vi "ScanMode.vi"() -> ()   [LabVIEW 2014]
uses:
  ScanDM.ctl
  MetricControl.ctl
  Scan Metric.ctl
  <vilib>/Analysis/6fits.llb/Curve Fitting Criteria.ctl
  ScanEngineState.ctl
  <vilib>/Utility/miscctls.llb/LVPointDoubleTypeDef.ctl
  <vilib>/Analysis/NI_AALPro.lvlib
  <vilib>/gmath/NI_Gmath.lvlib
panel:
  in  "parameter bounds":T1={"amp min"=-inf, "amp max"=inf, "center min"=-inf, "center max"=inf, "deviation min"=-inf, "deviation max"=inf, "offset min"=0.0, "offset max"=0.0}
  in  "tolerance":dbl=0.0001 format="%#_3g"
  out "Best Gaussian Fit":dbl[](array[numeric])
  in  "method":T2 items=["Least Square", "Least Absolute Residual", "Bisquare"]
  in  "Manual Initial Guess":bool
  in  "Initial Guess":T3={"initial amplitude"=nan, "initial center"=nan, "initial standard deviation"=nan, "offset"=nan}
  in  "Fit Type":enum32{"Guass Fit", "Quad Fit"}(radio)
  out "Intensity Graph":sgl[][](graph)
  in  "Apply":bool
  in  "Find peak":bool
  in  "Cancel":bool
  in  "Metric Control":T4={"Use Metric"=FALSE, "DM Metric"=enum."No Zero Mean", "Smooth"=FALSE, "Pixels"=0.0, "ROI"=FALSE, "ROI Size"=0.0}
  in  "stop":bool
  out "Metric Display":cluster{"Amplititude":dbl[], "Metric":sgl[]}[](graph)
  in  "Scan Control":T6 {"Mode" items=["1", "2", "3", "4", "5", "6", "7", "8", "9", "10", "11", "12", "13", "14", "15", "16", "17", "18", "19", "20", "21", "22", "23", "24", "25", "26", "27", "28", "29", "30", "31", "32", "33", "34", "35", "36", "37", "38", "39", "40", "41", "42", "43", "44", "45", "46", "47", "48", "49", "50", "51", "52", "53", "54", "55", "56", "57", "58", "59", "60", "61", "62", "63", "64", "65", "66", "67", "68", "69", "70", "71", "72", "73", "74", "75", "76", "77", "78", "79", "80", "81", "82", "83", "84", "85", "86", "87", "88", "89", "90", "91", "92", "93", "94", "95", "96", "97", "98", "99", "100", "101", "102", "103", "104", "105", "106", "107", "108", "109", "110", "111", "112", "113", "114", "115", "116", "117", "118", "119", "120", "121", "122", "123", "124", "125", "126", "127", "128", "129", "130", "131", "132", "133", "134", "135", "136", "137", "138", "139", "140"]}
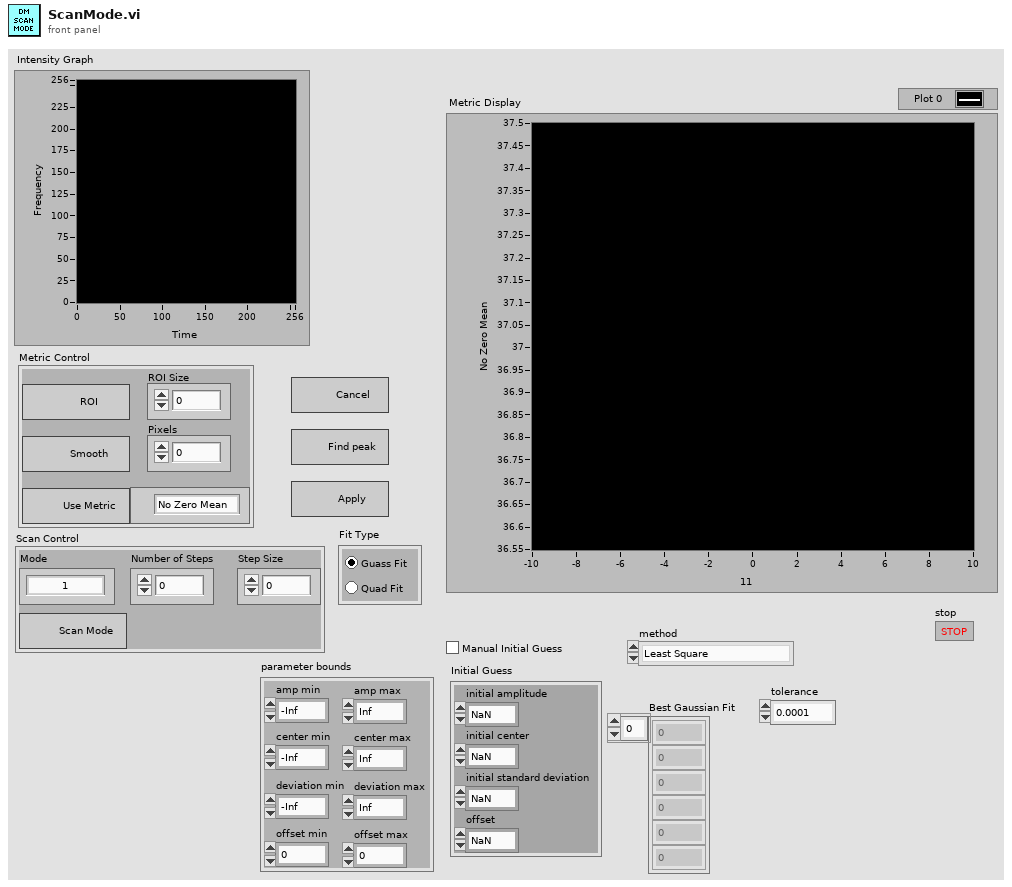
[diagram p1: front panel]
types:
  T1 = cluster{"amp min":dbl, "amp max":dbl, "center min":dbl, "center max":dbl, "deviation min":dbl, "deviation max":dbl, "offset min":dbl, "offset max":dbl}
  T2 = typedef "NI_AALPro.lvlib/Curve Fitting Criteria.ctl" = u16
  T3 = cluster{"initial amplitude":dbl, "initial center":dbl, "initial standard deviation":dbl, "offset":dbl}
  T4 = typedef "MetricControl.ctl" = cluster{"Use Metric":bool, "DM Metric":T5, "Smooth":bool, "Pixels":dbl, "ROI":bool, "ROI Size":dbl}
  T5 = typedef "Scan Metric.ctl" = enum16{"Max Intensity", "No Zero Mean", "Threshold"}
  T6 = typedef "ScanDM.ctl" = cluster{"Scan":bool, "Mode":u16, "Number of Steps":u8, "Step Size":dbl}
  T7 = typedef "ScanEngineState.ctl" = enum16{"DM_WRITE", "IMAGE", ""}
  T8 = typedef "LVPointDoubleTypeDef.ctl" = cluster{"X":dbl, "Y":dbl}
  T9 = enum16{"Linear", "Polynomial", "Exponential", "Power"}
  T10 = typedef "DMControl_STED.ctl" = cluster{"Type":enum32{"Mirror", "Abberation"}, "Modes":cluster{"Mode":string, "Amplititude":dbl}[], "Apply Flat":bool, "Save Map":bool, "Clear Voltage":bool, "Abberation Files":u16, "Scan ":bool}
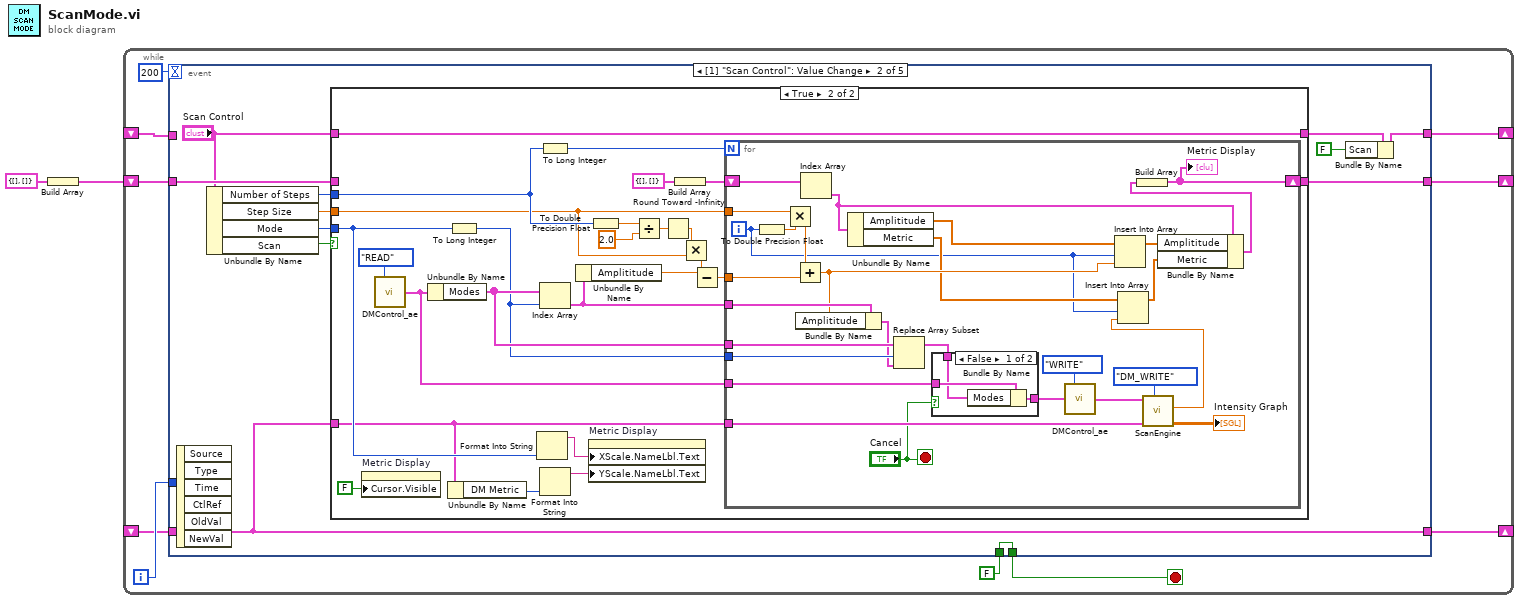
[diagram p0: block diagram]
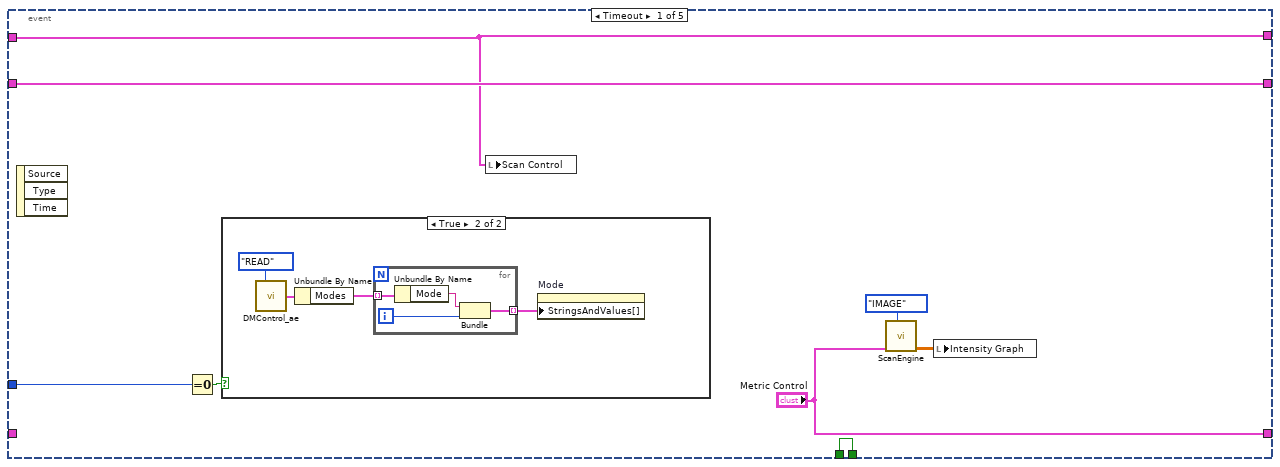
[diagram p2: hidden frame]
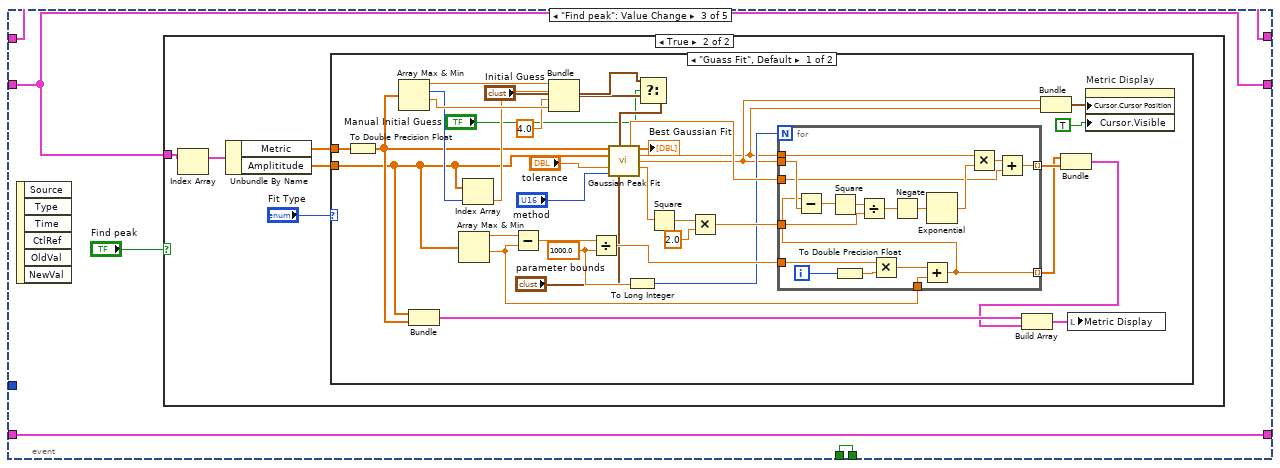
[diagram p6: hidden frame]
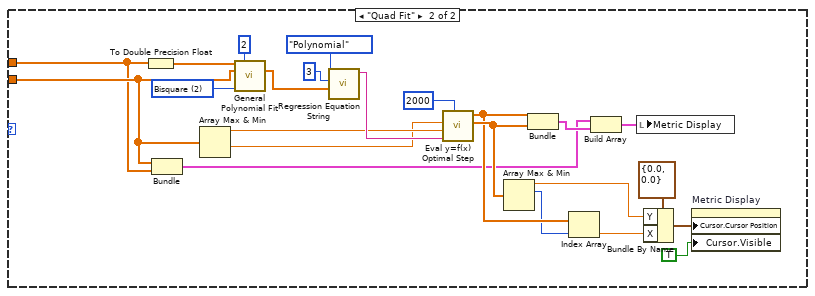
[diagram p8: hidden frame]
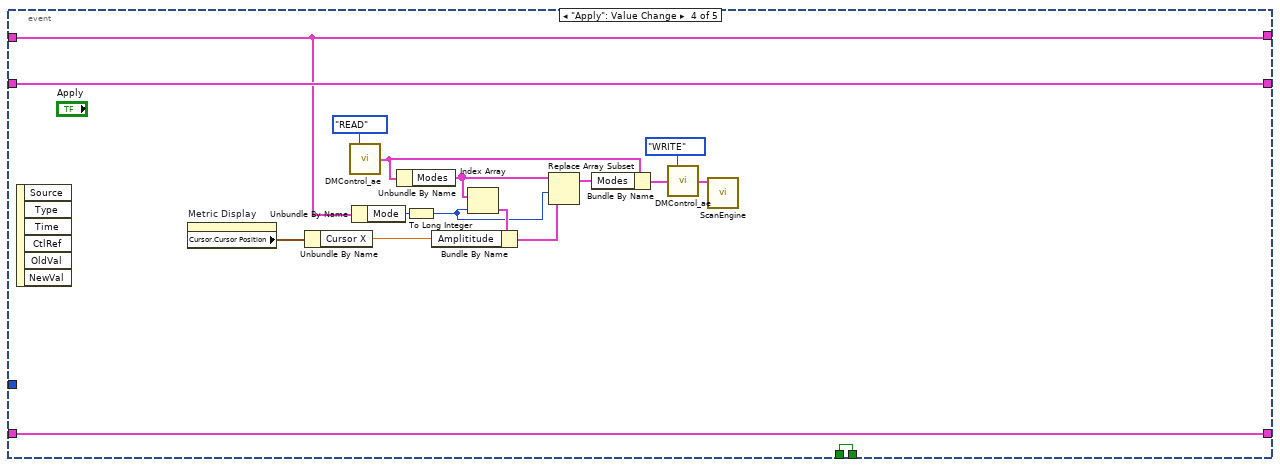
[diagram p9: hidden frame]
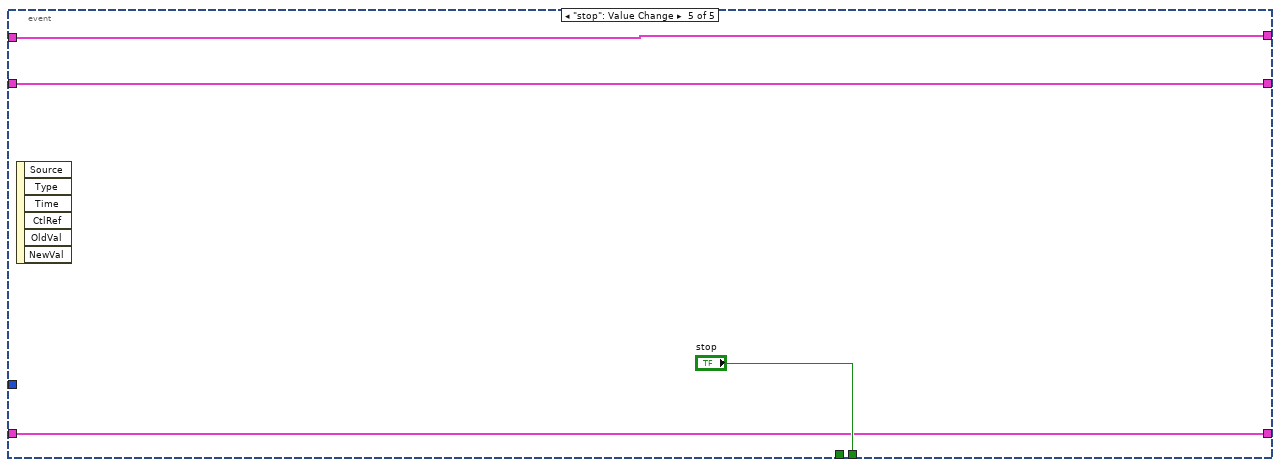
[diagram p10: hidden frame]
diagram:
  n1 = Build Array(cluster{"Amplititude":dbl[], "Metric":sgl[]} {"Amplititude"=[], "Metric"=[]} ("output cluster")) -> (w1:cluster{"Amplititude":dbl[], "Metric":sgl[]}[])
  n2 = while {
    shift-right: [w8] -> _
    shift-left: _ -> [w7]
    shift-right: [w6] -> _
    shift-left: w1 -> [w5]
    shift-right: [w3] -> _
    shift-left: _ -> [w4]
    i -> [w9]
    stop <- w12 stop-if-true
    n3 = event shown="[1] \"Scan Control\": Value Change" {
      selector: _ -> [_ _ _ _ _]
      dyn-events: _ -> [_ _ _ _ _]
      timeout: 200 -> [_ _ _ _ _]
      tunnel: [w20 w38 w101 w187 "stop"] -> w12
      tunnel: FALSE -> [w20 w38 w101 w187 _]
      tunnel: w9 -> [w18 _ _ _ _]
      tunnel: [w16 w30 w104 w198 w205] -> w8
      tunnel: w7 -> [w16 _ w104 w198 w205]
      tunnel: [w17 w36 w103 w202 w204] -> w6
      tunnel: w5 -> [w17 w34 w103 w202 w204]
      tunnel: w4 -> [_ w29 w100 w186 w203]
      tunnel: ["Metric Control" w29 w100 w186 w203] -> w3
      event Timeout {
        n4 = event-data() -> ()  [unwired: 1 in, 3 out]
        n5 = Equal To 0?(x=w18) -> (x = 0?=w19:bool)
        n6 = case shown="True" w19 {
          frame False {
          }
          frame True {
            n7 = call "DMControl_ae.vi"("Enum"=enum16{"WRITE", "READ"}."READ") -> ("Abberation Cluster Out"=w23:T10)  [unwired: 14 in]
            n8 = Unbundle By Name(w23) -> ("Modes"=w22:cluster{"Mode":string, "Amplititude":dbl}[])
            n9 = for {
              tunnel: w22 -> [w28] mode=indexing
              tunnel: [w25] -> w21 mode=indexing
              i -> [w26]
              n10 = Unbundle By Name(w28) -> ("Mode"=w27:string)
              n11 = Bundle("Mode"=w27, w26) -> (w25:cluster{"Mode":string, i32})  [unwired: 1 in]
            }
            n12 = property on="Mode" class="Ring (strict)"("StringsAndValues[]"=w21) -> ()  [unwired: 2 in, 2 out]
          }
        }
        n13 = local write "Scan Control"(w16) -> ()
        n14 = call "ScanEngine.vi"("Action"=ScanEngineState."IMAGE", "Metric Control"="Metric Control") -> ("Metric Image"=w13:sgl[][])  [unwired: 8 in, 1 out]
        n15 = local write "Intensity Graph"(w13) -> ()
      }
      event Value Change {
        n16 = event-data() -> ()  [unwired: 1 in, 6 out]
        n17 = Unbundle By Name("Scan Control") -> ("Number of Steps"=w40:u8, "Step Size"=w39:dbl, "Mode"=w37:u16, "Scan"=w35:bool)
        n18 = case shown="True" w35 {
          tunnel: w40 -> [_ w62]
          tunnel: w39 -> [_ w61]
          tunnel: w37 -> [_ w50]
          tunnel: [w42 w44] -> w36
          tunnel: w34 -> [w42 _]
          tunnel: [w41 w48] -> w31
          tunnel: "Scan Control" -> [w41 w48]
          tunnel: w29 -> [_ w43]
          frame False {
          }
          frame True {
            n19 = property on="Metric Display" class="XYGraph (strict)"("Cursor.Visible"=FALSE) -> ()  [unwired: 2 in, 2 out]
            n20 = call "DMControl_ae.vi"("Enum"=enum16{"WRITE", "READ"}."READ") -> ("Abberation Cluster Out"=w54:T10)  [unwired: 14 in]
            n21 = Unbundle By Name(w54) -> ("Modes"=w56:cluster{"Mode":string, "Amplititude":dbl}[])
            n22 = Unbundle By Name(w43) -> ("DM Metric"=w49:T5)
            n23 = To Long Integer(number=w50) -> (32bit integer=w55:i32)
            n24 = Format Into String(w50) -> (resulting string=w51:string)  [unwired: 3 in, 1 out]
            n25 = To Long Integer(number=w62) -> (32bit integer=w53:i32)
            n26 = Index Array(array=w56, index=w55) -> (element=w57:cluster{"Mode":string, "Amplititude":dbl})
            n27 = Format Into String(w49) -> (resulting string=w52:string)  [unwired: 3 in, 1 out]
            n28 = Unbundle By Name(w57) -> ("Amplititude"=w60:dbl)
            n29 = property on="Metric Display" class="XYGraph (strict)"("XScale.NameLbl.Text"=w51, "YScale.NameLbl.Text"=w52) -> ()  [unwired: 2 in, 2 out]
            n30 = To Double Precision Float(number=w62) -> (double precision float=w63:dbl)
            n31 = Divide(x=w63, y=2.0) -> (x/y=w65:dbl)
            n32 = Round Toward -Infinity(1:w65) -> (0:w66:dbl)
            n33 = Build Array(cluster{"Amplititude":dbl[], "Metric":sgl[]} {"Amplititude"=[], "Metric"=[]} ("output cluster")) -> (w45:cluster{"Amplititude":dbl[], "Metric":sgl[]}[])
            n34 = Multiply(x=w66, y=w61) -> (x*y=w59:dbl)
            n35 = Subtract(x=w60, y=w59) -> (x-y=w58:dbl)
            n36 = for {
              N: w53 -> [_]
              tunnel: w61 -> [w95]
              tunnel: w58 -> [w94]
              tunnel: w57 -> [w93]
              tunnel: w56 -> [w92]
              tunnel: w55 -> [w91]
              tunnel: w54 -> [w90]
              shift-right: [w70] -> w44
              shift-left: w45 -> [w80]
              tunnel: w43 -> [w89]
              i -> [w76]
              stop <- "Cancel" stop-if-true
              n37 = To Double Precision Float(number=w76) -> (double precision float=w88:dbl)
              n38 = Multiply(x=w95, y=w88) -> (x*y=w87:dbl)
              n39 = Add(x=w87, y=w94) -> (x+y=w78:dbl)
              n40 = Bundle By Name(cluster=w93, "Amplititude"=w78) -> (w86:cluster{"Mode":string, "Amplititude":dbl})
              n41 = Index Array(array=w80) -> (element=w74:cluster{"Amplititude":dbl[], "Metric":sgl[]})  [unwired: 1 in]
              n42 = Unbundle By Name(w74) -> ("Amplititude"=w79:dbl[], "Metric"=w77:sgl[])
              n43 = Replace Array Subset(array=w92, new element=w86, index=w91) -> (w83:cluster{"Mode":string, "Amplititude":dbl}[])
              n44 = case shown="False" "Cancel" {
                tunnel: w90 -> [w98 w99]
                tunnel: [w97 w99] -> w84
                tunnel: w83 -> [w96 _]
                frame False {
                  n45 = Bundle By Name(cluster=w98, "Modes"=w96) -> (w97:T10)
                }
                frame True {
                }
              }
              n46 = call "DMControl_ae.vi"("Enum"=enum16{"WRITE", "READ"}."WRITE", "Control"=w84) -> ("Abberation Cluster Out"=w82:T10)  [unwired: 13 in]
              n47 = Insert Into Array(array=w79, index=w76, new element=w78) -> (w73:dbl[])
              n48 = call "ScanEngine.vi"("Action"=ScanEngineState."DM_WRITE", "Metric Control"=w89, "Abberation Cluster"=w82) -> ("Metric Image"=→"Intensity Graph":sgl[][], "Metric Result"=w75:dbl)  [unwired: 7 in]
              n49 = Insert Into Array(array=w77, index=w76, new element=w75) -> (w72:sgl[])
              n50 = Bundle By Name(cluster=w74, "Amplititude"=w73, "Metric"=w72) -> (w71:cluster{"Amplititude":dbl[], "Metric":sgl[]})
              n51 = Build Array(w71) -> (w70:cluster{"Amplititude":dbl[], "Metric":sgl[]}[])
              "Metric Display" <- w70
            }
          }
        }
        n52 = Bundle By Name(cluster=w31, "Scan"=FALSE) -> (w30:T6)
      }
      event "Find peak": Value Change {
        n53 = event-data() -> ()  [unwired: 1 in, 6 out]
        n54 = case shown="True" "Find peak" {
          tunnel: w103 -> [_ w107]
          frame False {
          }
          frame True {
            n55 = Index Array(array=w107) -> (element=w106:cluster{"Amplititude":dbl[], "Metric":sgl[]})  [unwired: 1 in]
            n56 = Unbundle By Name(w106) -> ("Metric"=w108:sgl[], "Amplititude"=w109:dbl[])
            n57 = case shown="\"Guass Fit\", Default" "Fit Type" {
              tunnel: w109 -> [w128 w167]
              tunnel: w108 -> [w144 w166]
              frame "Guass Fit", Default {
                w122 = 1000.0 ("y")
                n58 = To Double Precision Float(number=w144) -> (double precision float=w133:dbl[])
                n59 = Array Max & Min(array=w133) -> (max value=w143:dbl, max index (indices)=w140:i32, min value=w142:dbl)  [unwired: 1 out]
                n60 = Bundle("Amplititude"=w128, w133) -> (w132:cluster{"Amplititude":dbl[], dbl[]})  [unwired: 1 in]
                n61 = Array Max & Min(array=w128) -> (max value=w127:dbl, min value=w124:dbl)  [unwired: 2 out]
                n62 = Index Array(array=w128, index=w140) -> (element=w139:dbl)
                n63 = Subtract(x=w127, y=w124) -> (x-y=w126:dbl)
                n64 = Bundle(w143, w139, 4.0, w142) -> (w115:cluster{dbl, dbl, dbl, dbl})  [unwired: 1 in]
                n65 = Divide(x=w126, y=w122) -> (x/y=w125:dbl)
                n66 = To Long Integer(number=w122) -> (32bit integer=w121:i32)
                n67 = Select(t="Initial Guess", s="Manual Initial Guess", f=w115) -> (s? t:f=w114:T3)
                n68 = call <vilib>:"Gaussian Peak Fit.vi"("Y"=w133, "initial guess"=w114, "X"=w128, "tolerance"="tolerance", "method"="method", "parameter bounds"="parameter bounds") -> ("offset"=w130:dbl, "Best Gaussian Fit"=→"Best Gaussian Fit":dbl[], "amplitude"=w117:dbl, "center"=w118:dbl, "standard deviation"=w129:dbl)  [unwired: 3 in, 2 out]
                n69 = Square(x=w129) -> (x^2=w138:dbl)
                n70 = Multiply(x=w138, y=2.0) -> (x*y=w136:dbl)
                n71 = for {
                  N: w121 -> [_]
                  tunnel: w117 -> [w162]
                  tunnel: w118 -> [w161]
                  tunnel: w130 -> [w153]
                  tunnel: w136 -> [w158]
                  tunnel: [w152] -> w134 mode=indexing
                  tunnel: w125 -> [w149]
                  tunnel: w124 -> [w147]
                  tunnel: [w146] -> w123 mode=indexing
                  i -> [w151]
                  n72 = To Double Precision Float(number=w151) -> (double precision float=w150:dbl)
                  n73 = Multiply(x=w149, y=w150) -> (x*y=w148:dbl)
                  n74 = Add(x=w148, y=w147) -> (x+y=w146:dbl)
                  n75 = Subtract(x=w146, y=w161) -> (x-y=w160:dbl)
                  n76 = Square(x=w160) -> (x^2=w159:dbl)
                  n77 = Divide(x=w159, y=w158) -> (x/y=w157:dbl)
                  n78 = Negate(x=w157) -> (-x=w156:dbl)
                  n79 = Exponential(1:w156) -> (0:w155:dbl)
                  n80 = Multiply(x=w162, y=w155) -> (x*y=w154:dbl)
                  n81 = Add(x=w154, y=w153) -> (x+y=w152:dbl)
                }
                n82 = Bundle("center"=w118, "amplitude"=w117) -> (w120:cluster{"center":dbl, "amplitude":dbl})  [unwired: 1 in]
                n83 = Bundle(w123, w134) -> (w131:cluster{dbl[], dbl[]})  [unwired: 1 in]
                n84 = Build Array(w132, w131) -> (w135:cluster{"Amplititude":dbl[], dbl[]}[])
                n85 = local write "Metric Display"(w135) -> ()
                n86 = property on="Metric Display" class="XYGraph (strict)"("Cursor.Cursor Position"=w120, "Cursor.Visible"=TRUE) -> ()  [unwired: 2 in, 2 out]
              }
              frame "Quad Fit" {
                w184 = T2 2 items=["Least Square", "Least Absolute Residual", "Bisquare"] ("method")
                n87 = To Double Precision Float(number=w166) -> (double precision float=w185:dbl[])
                n88 = Bundle("Amplititude"=w167, "Metric"=w166) -> (w163:cluster{"Amplititude":dbl[], "Metric":sgl[]})  [unwired: 1 in]
                n89 = Array Max & Min(array=w167) -> (max value=w177:dbl, min value=w176:dbl)  [unwired: 2 out]
                n90 = call <vilib>:"General Polynomial Fit.vi"("Y"=w185, "polynomial order"=2, "X"=w167, "method"=w184) -> ("Polynomial Coefficients"=w181:dbl[])  [unwired: 8 in, 3 out]
                n91 = call "Regression Equation String.vi"("coefficients"=w181, "precision"=3, "fit type"=T9."Polynomial") -> ("Formula"=w179:string)  [unwired: 8 in]
                n92 = call <vilib>:"Eval y=f(x) Optimal Step.vi"("number of points"=u32 2000, "formula"=w179, "end"=w177, "start"=w176) -> ("Y Values"=w175:dbl[], "X Values"=w174:dbl[])  [unwired: 1 in, 2 out]
                n93 = Array Max & Min(array=w175) -> (max value=w171:dbl, max index (indices)=w173:i32)  [unwired: 2 out]
                n94 = Bundle("X Values"=w174, "Y Values"=w175) -> (w164:cluster{"X Values":dbl[], "Y Values":dbl[]})  [unwired: 1 in]
                n95 = Index Array(array=w174, index=w173) -> (element=w170:dbl)
                n96 = Build Array(w163, w164) -> (w165:cluster{"X Values":dbl[], "Y Values":dbl[]}[])
                n97 = local write "Metric Display"(w165) -> ()
                n98 = Bundle By Name(cluster=T8 {"X"=0.0, "Y"=0.0} ("Cursor.Cursor Position"), "Y"=w171, "X"=w170) -> (w169:T8)
                n99 = property on="Metric Display" class="XYGraph (strict)"("Cursor.Cursor Position"=w169, "Cursor.Visible"=TRUE) -> ()  [unwired: 2 in, 2 out]
              }
            }
          }
        }
      }
      event "Apply": Value Change {
        n100 = event-data() -> ()  [unwired: 1 in, 6 out]
        n101 = property on="Metric Display" class="XYGraph (strict)"() -> ("Cursor.Cursor Position"=w201:T8)  [unwired: 2 in, 2 out]
        n102 = Unbundle By Name(w201) -> ("Cursor X"=w194:dbl)
        n103 = call "DMControl_ae.vi"("Enum"=enum16{"WRITE", "READ"}."READ") -> ("Abberation Cluster Out"=w190:T10)  [unwired: 14 in]
        n104 = Unbundle By Name(w198) -> ("Mode"=w196:u16)
        n105 = Unbundle By Name(w190) -> ("Modes"=w192:cluster{"Mode":string, "Amplititude":dbl}[])
        n106 = To Long Integer(number=w196) -> (32bit integer=w193:i32)
        n107 = Index Array(array=w192, index=w193) -> (element=w195:cluster{"Mode":string, "Amplititude":dbl})
        n108 = Bundle By Name(cluster=w195, "Amplititude"=w194) -> (w191:cluster{"Mode":string, "Amplititude":dbl})
        n109 = Replace Array Subset(array=w192, new element=w191, index=w193) -> (w189:cluster{"Mode":string, "Amplititude":dbl}[])
        n110 = Bundle By Name(cluster=w190, "Modes"=w189) -> (w188:T10)
        n111 = call "DMControl_ae.vi"("Enum"=enum16{"WRITE", "READ"}."WRITE", "Control"=w188) -> ("Abberation Cluster Out"=w199:T10)  [unwired: 13 in]
        n112 = call "ScanEngine.vi"("Abberation Cluster"=w199) -> ()  [unwired: 9 in, 2 out]
      }
      event "stop": Value Change {
        n113 = event-data() -> ()  [unwired: 1 in, 6 out]
      }
    }
  }
